vi "18.OCR.vi"() -> ()   [LabVIEW 2017]
uses:
  <vilib>/userdefined/High Color/IMAQdx.ctl
  <vilib>/vision/OCR.llb/IMAQ OCR Character Report 2.ctl
  <vilib>/vision/driver/NI_Vision_Acquisition_Software.lvlib
  <vilib>/vision/NI_Vision_Development_Module.lvlib
panel:
  out "Character Reports":T1[](array[typedef]) {"Character Statistics"."Threshold Range"."Upper value" format="%.2f"; "Character Statistics"."Threshold Range"."Lower value" format="%.2f"}
  out "Image Out":T2(plugin-control)
  out "error out":errorcluster
  out "String (OCR)":string
  out "Image Local Average":T2(plugin-control)
  in  "Camera Select":T3
  in  "停止":bool
  out "Image In":T2(plugin-control)
  out "Image Threshold":T2(plugin-control)
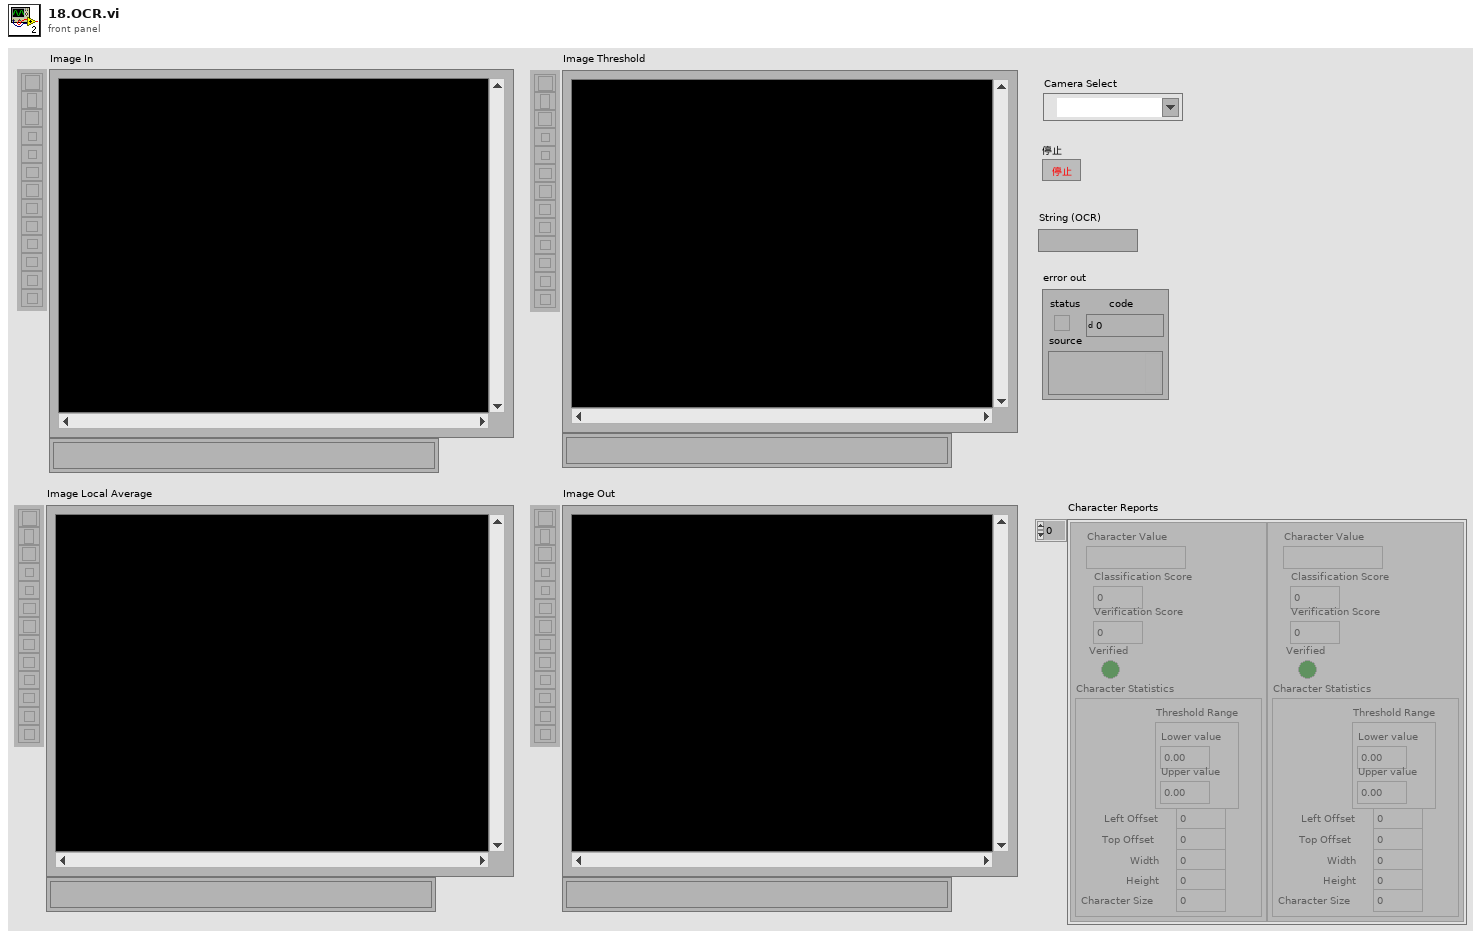
[diagram p1: front panel]
types:
  T1 = typedef "IMAQ OCR Character Report 2.ctl" = cluster{"Character Value":string, "Classification Score":i32, "Verification Score":i32, "Verified":bool, "Character Statistics":cluster{"Threshold Range":cluster{"Lower value":sgl, "Upper value":sgl}, "Left Offset":i32, "Top Offset":i32, "Width":i32, "Height":i32, "Character Size":i32}}
  T2 = typedef "IMAQ Image.ctl" = refnum<image>
  T3 = typedef "IMAQdx.ctl" = refnum<k21>
  T4 = enum32{"AutoM", "Close", "Dilate", "Erode", "Gradient", "Gradient out", "Gradient in", "Hit miss", "Open", "PClose", "POpen", "Thick", "Thin"}
  T5 = cluster{"Threshold Data":cluster{"Method":enum16{"Fixed Range", "Uniform", "Linear", "Non Linear", "Local", "Color"}, "Looking for":u32, "Color Mode":u32, "Kernel Size":cluster{"Width":i32, "Height":i32}, "Ranges":cluster{"Min":i32, "Max":i32}[]}, "Reject Border":bool, "Number Of Erosions":i32, "Size & Spacing":cluster{"Segment Algorithm":u16, "Min Bounding Rect Width":i32, "Max Bounding Rect Width":i32, "Min Bounding Rect Height":i32, "Max Bounding Rect Height":i32, "Min Character Size":i32, "Max Character Size":i32, "Min Char Spacing":i32, "Max Horiz Element Spacing":i32, "Max Vert Element Spacing":i32, "Max Space Distance":i32}, "Read Options":cluster{"Read Strategy":i32, "Read Resolution":i32, "Scale Dependant":bool, "Aspect Ratio":i32, "Acceptance Level":i32, "Substitution Character":string, "MultiLine":bool}, "Valid Characters":cluster{"Pre-defined characters":i32, "User-defined characters":string}[], "Use Text Pattern":bool, "Orientation":u32, "# Lines Expected":u32, "Number of Blocks":i32}
  T6 = cluster{"Global Rectangle":i32[], "Contours":cluster{"ID":enum32{"External", "Internal"}, "Type":u32, "Coordinates":i32[]}[]}
  T7 = typedef "IMAQ OCR Session.ctl" = refnum<k1>
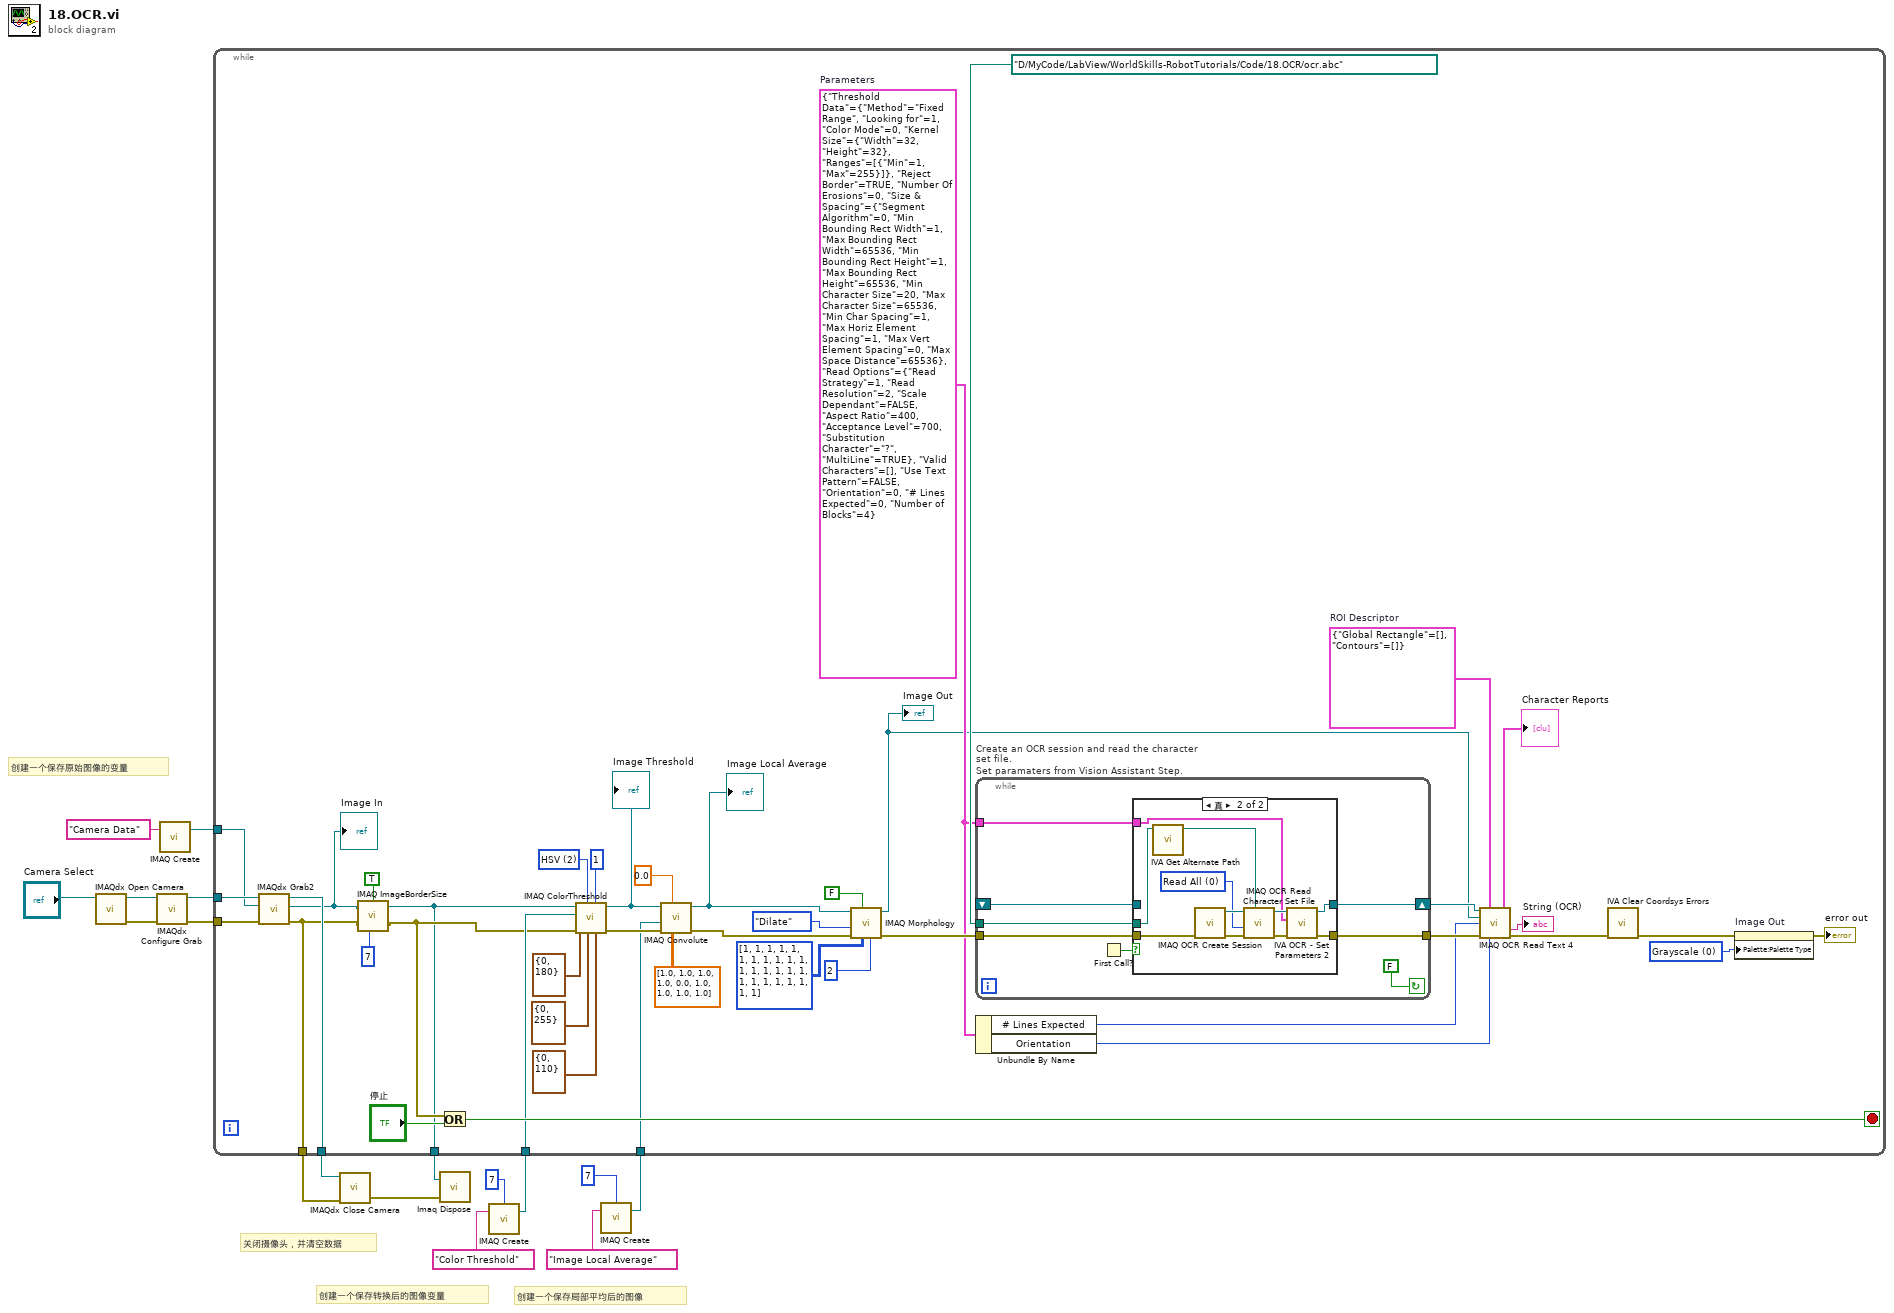
[diagram p0: block diagram]
diagram:
  # "创建一个保存局部平均后的图像"
  # "创建一个保存原始图像的变量"
  # "创建一个保存转换后的图像变量"
  # "关闭摄像头，并清空数据"
  n1 = call <vilib>:"IMAQdx Open Camera.vi"("Session In"="Camera Select") -> ("error out"=w17:errorcluster, "Session Out"=w16:T3)  [unwired: 9 in]
  n2 = call <vilib>:"IMAQdx Configure Grab.vi"("error in"=w17, "Session In"=w16) -> ("error out"=w14:errorcluster, "Session Out"=w15:T3)  [unwired: 8 in]
  n3 = call "IMAQ Create"("Image Name"="Camera Data") -> ("New Image"=w13:T2)  [unwired: 4 in, 1 out]
  n4 = call "IMAQ Create"("Border Size"=7, "Image Name"="Color Threshold") -> ("New Image"=w6:T2)  [unwired: 3 in, 1 out]
  n5 = call "IMAQ Create"("Border Size"=7, "Image Name"="Image Local Average") -> ("New Image"=w3:T2)  [unwired: 3 in, 1 out]
  n6 = while {
    tunnel: w15 -> [w61]
    tunnel: w14 -> [w60]
    tunnel: w13 -> [w59]
    tunnel: [w50] -> w10
    tunnel: [w48] -> w9
    tunnel: [w44] -> w7
    tunnel: w6 -> [w51]
    tunnel: w3 -> [w39]
    stop <- w53 stop-if-true
    w21 = u32 0 items=["Grayscale", "Binary", "Gradient", "Rainbow", "Temperature", "User Defined", "Binary 16 Bit", "Gradient 16 Bit", "Rainbow 16 Bit", "Temperature 16 Bit", "User Defined 16 Bit"] ("Palette Type")
    w30 = T5 {"Threshold Data"={"Method"=enum."Fixed Range", "Looking for"=1, "Color Mode"=0, "Kernel Size"={"Width"=32, "Height"=32}, "Ranges"=[{"Min"=1, "Max"=255}]}, "Reject Border"=TRUE, "Number Of Erosions"=0, "Size & Spacing"={"Segment Algorithm"=0, "Min Bounding Rect Width"=1, "Max Bounding Rect Width"=65536, "Min Bounding Rect Height"=1, "Max Bounding Rect Height"=65536, "Min Character Size"=20, "Max Character Size"=65536, "Min Char Spacing"=1, "Max Horiz Element Spacing"=1, "Max Vert Element Spacing"=0, "Max Space Distance"=65536}, "Read Options"={"Read Strategy"=1, "Read Resolution"=2, "Scale Dependant"=FALSE, "Aspect Ratio"=400, "Acceptance Level"=700, "Substitution Character"="?", "MultiLine"=TRUE}, "Valid Characters"=[], "Use Text Pattern"=FALSE, "Orientation"=0, "# Lines Expected"=0, "Number of Blocks"=4}  # Parameters
    w32 = T6 {"Global Rectangle"=[], "Contours"=[]}  # ROI Descriptor
    w57 = u16 2 items=["RGB", "HSL", "HSV", "HSI"] ("Color Mode")
    n7 = call <vilib>:"IMAQdx Grab2.vi"("error in"=w60, "Image In"=w59, "Session In"=w61) -> ("error out"=w48:errorcluster, "Image Out"=w49:T2, "Session Out"=w50:T3)  [unwired: 5 in, 1 out]
    "Image In" <- w49
    n8 = call "IMAQ ImageBorderSize"("Get/Set Status? (Set)"=TRUE, "Image"=w49, "Image border size in"=7, "error in (no error)"=w48) -> ("Image Out"=w44:T2, "error out"=w45:errorcluster)  [unwired: 1 out]
    n9 = Or(x=w45, y="停止") -> (x .or. y?=w53:bool)
    n10 = call "IMAQ ColorThreshold"("Blue or Luma or Val or Inten Range"=cluster{"Lower value":i32, "Upper value":i32} {"Lower value"=0, "Upper value"=110}, "Replace Value"=1, "Green or Sat Range"=cluster{"Lower value":i32, "Upper value":i32} {"Lower value"=0, "Upper value"=255}, "Color Mode"=w57, "error in (no error)"=w45, "Red or Hue Range"=cluster{"Lower value":i32, "Upper value":i32} {"Lower value"=0, "Upper value"=180}, "Image Dst"=w51, "Image Src"=w44) -> ("error out"=w42:errorcluster, "Image Dst Out"=w43:T2)  [unwired: 2 out]
    "Image Threshold" <- w43
    n11 = call "IMAQ Convolute"("Kernel"=sgl[][] [[1.0, 1.0, 1.0], [1.0, 0.0, 1.0], [1.0, 1.0, 1.0]], "Divider (kernel sum)"=sgl 0.0, "error in (no error)"=w42, "Image Dst"=w39, "Image Src"=w43) -> ("error out"=w19:errorcluster, "Image Dst Out"=w20:T2)  [unwired: 2 in, 3 out]
    "Image Local Average" <- w20
    n12 = call "IMAQ Morphology"("Number of iterations (1)"=2, "Structuring Element"=i32[][] [[1, 1, 1, 1, 1], [1, 1, 1, 1, 1], [1, 1, 1, 1, 1], [1, 1, 1, 1, 1], [1, 1, 1, 1, 1]], "Square/Hexa (Square)"=FALSE, "error in (no error)"=w19, "Operation"=T4."Dilate", "Image Src"=w20) -> ("error out"=w31:errorcluster, "Image Dst Out"=w22:T2)  [unwired: 1 in, 3 out]
    "Image Out" <- w22
    n13 = while "Create an OCR session and read the character set file.\nSet paramaters from Vision Assistant Step." {
      shift-right: [w66] -> w28
      shift-left: _ -> [w65]
      tunnel: w31 -> [w68]
      tunnel: w30 -> [w64]
      tunnel: path "D:/MyCode/LabView/WorldSkills-RobotTutorials/Code/18.OCR/ocr.abc" ("File Path") -> [w63]
      tunnel: [w62] -> w29
      stop <- FALSE continue-if-true
      n14 = First Call?() -> (First Call?: T/F=w67:bool)
      n15 = case "条件结构" shown="真" w67 {
        tunnel: w63 -> [_ w75]
        tunnel: w68 -> [w70 w79]
        tunnel: [w71 w77] -> w66
        tunnel: [w70 w76] -> w62
        tunnel: w64 -> [_ w72]
        tunnel: w65 -> [w71 _]
        frame False {
        }
        frame True {
          w80 = 0 items=["Read All", "Read Character Set Only", "Read Properties Only"] ("Read Options")
          n16 = call <vilib>:"IVA Get Alternate Path.vi"("Path In"=w75) -> ("Path Out"=w74:path)  [unwired: 10 out]
          n17 = call "IMAQ OCR Create Session"("error in (no error)"=w79) -> ("error out"=w81:errorcluster, "IMAQ OCR Session"=w82:T7)  [unwired: 9 out]
          n18 = call "IMAQ OCR Read Character Set File"("File Path"=w74, "error in (no error)"=w81, "Read Options"=w80, "IMAQ OCR Session"=w82) -> ("error out"=w78:errorcluster, "IMAQ OCR Session (dup)"=w73:T7)  [unwired: 1 in, 5 out]
          n19 = call <vilib>:"IVA OCR - Set Parameters 2.vi"("error in (no error)"=w78, "Parameters"=w72, "IMAQ OCR Session"=w73) -> ("error out"=w76:errorcluster, "IMAQ OCR Session Out"=w77:T7)  [unwired: 7 in]
        }
      }
    }
    n20 = Unbundle By Name(w30) -> ("# Lines Expected"=w26:u32, "Orientation"=w27:u32)
    n21 = call "IMAQ OCR Read Text 4"("IMAQ OCR Session"=w28, "ROI Descriptor"=w32, "Image"=w22, "Number of Lines Requested"=w26, "error in (no error)"=w29, "Orientation"=w27) -> ("Character Reports"=→"Character Reports":T1[], "Read String"=→"String (OCR)":string, "error out"=w25:errorcluster)  [unwired: 7 out]
    n22 = call <vilib>:"IVA Clear Coordsys Errors.vi"("error in (no error)"=w25) -> ("error out"=w24:errorcluster)  [unwired: 10 in]
    n23 = property on="Image Out" class="ImageControl"(error in=w24, "Palette:Palette Type"=w21) -> (error out=→"error out":errorcluster)  [unwired: 1 in, 1 out]
  }
  n24 = call <vilib>:"IMAQdx Close Camera.vi"("error in"=w9, "Session In"=w10) -> ("error out"=w8:errorcluster)  [unwired: 9 in]
  n25 = call "Imaq Dispose"("Image"=w7, "error in (no error)"=w8) -> ()  [unwired: 4 in, 1 out]
